vi "Read.EngineData.vi"(8 "error in":errorcluster, 11 "Read in":refnum<class "Read.lvclass">) -> (0 "error out":errorcluster, 3 "Read out":refnum<class "Read.lvclass">)   [LabVIEW 2023, in "Plugin Data Access Engine.lvlib" / "Read.lvclass"]
uses:
  Read.lvclass
  Read.lvclass/Read.ctl
  <vilib>/NI VeriStand/Custom Device API/Global Data Refs.vi
  <userlib>/PluginCore.lvlibp/iPluginAPIs/iPluginAPIs.lvclass
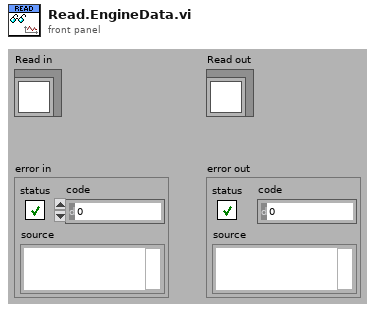
[diagram p1: front panel]
types:
  T1 = typedef "Custom Device API.lvlib/Block Data Reference.ctl" = cluster{"Data Reference":T2, "Offset":u64, "Length":u64}
  T2 = typedef "Custom Device API.lvlib/Data Reference.ctl" = i32
  T3 = cluster{"Data Reference":i32, "Offset":u64, "Length":u64}[]
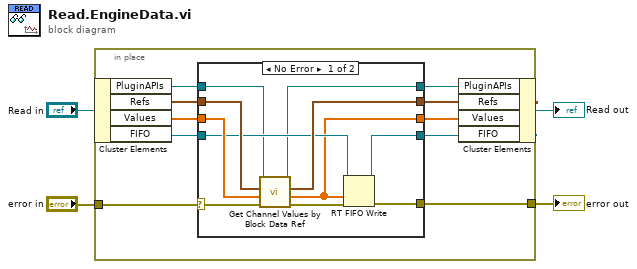
[diagram p0: block diagram]
diagram:
  n1 = in-place {
    in-place-border: [w14] -> w4
    in-place-border: "error in" -> [w11]
    n2 = in-place-cluster #1("Read in") -> ("PluginAPIs"=w6:refnum<class "iPluginAPIs.lvclass">, "Refs"=w13:T1[], "Values"=w10:dbl[], "FIFO"=w8:refnum<k33>)
    n3 = case shown="No Error" w11 {
      selector: w11 -> [w24 w30]
      tunnel: [w25 w30] -> w14
      tunnel: [w17 w28] -> w9
      tunnel: w13 -> [w22 w29]
      tunnel: [w21 w29] -> w12
      tunnel: w10 -> [w20 w28]
      tunnel: w8 -> [w19 w27]
      tunnel: [w18 w27] -> w7
      tunnel: w6 -> [w16 w26]
      tunnel: [w15 w26] -> w5
      frame No Error {
        n4 = call-dynamic "Get Channel Values by Block Data Ref.vi"("error in"=w24, "Values in"=w20, "Block Data Ref in"=w22, "iPluginAPI in"=w16) -> ("error out"=w23:errorcluster, "Values out"=w17:dbl[], "Block Data Ref out"=w21:T3, "iPluginAPI out"=w15:refnum<class "iPluginAPIs.lvclass">)  [unwired: 4 in]
        n5 = RT FIFO Write(0:w19, 1:w17, 3:w23) -> (8:w18:refnum<k33>, 11:w25:errorcluster)  [unwired: 2 in, 2 out]
      }
      frame Error {
      }
    }
    n6 = in-place-cluster #1("PluginAPIs"=w5, "Refs"=w12, "Values"=w9, "FIFO"=w7) -> (→"Read out":refnum<class "Read.lvclass">)
  }
  "error out" <- w4
